vi "Split Bank DIO.vi"(0 "IN 19:0":fxp<+,20,20> format="%.0b") -> (2 "OUT 1:0":fxp<+,2,2>, 3 "OUT 3:2":fxp<+,2,2>, 4 "OUT 7:4":fxp<+,4,4>, 6 "OUT 9:8":fxp<+,2,2>, 8 "OUT 11:10":fxp<+,2,2>, 10 "OUT 13:12":fxp<+,2,2>, 13 "OUT 19:18":fxp<+,2,2>, 14 "OUT 17:16":fxp<+,2,2>, 15 "OUT 15:14":fxp<+,2,2>)   [LabVIEW 2021]
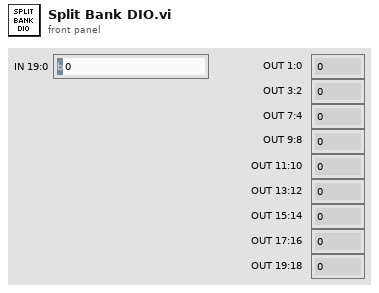
[diagram p1: front panel]
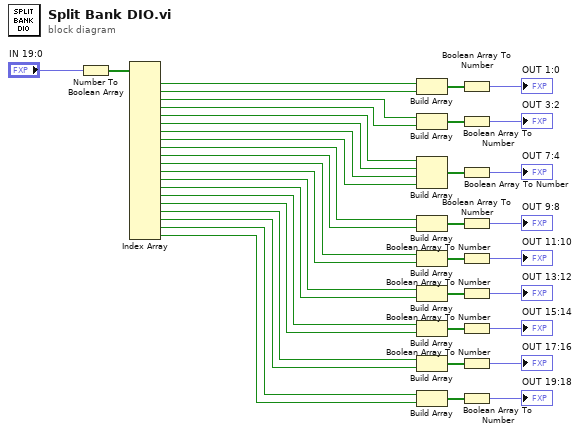
[diagram p0: block diagram]
diagram:
  n1 = Number To Boolean Array(number="IN 19:0") -> (Boolean array=w39:bool[])
  n2 = Index Array(array=w39) -> (element #1=w20:bool, element #2=w19:bool, element #3=w18:bool, element #4=w17:bool, element #5=w16:bool, element #6=w15:bool, element #7=w14:bool, element #8=w13:bool, element #9=w12:bool, element #10=w11:bool, element #11=w10:bool, element #12=w9:bool, element #13=w8:bool, element #14=w7:bool, element #15=w6:bool, element #16=w5:bool, element #17=w4:bool, element #18=w3:bool, element #19=w2:bool, element #20=w1:bool)  [unwired: 20 in]
  n3 = Build Array(w20, w19) -> (w38:bool[])
  n4 = Build Array(w18, w17) -> (w36:bool[])
  n5 = Build Array(w16, w15, w14, w13) -> (w35:bool[])
  n6 = Build Array(w12, w11) -> (w34:bool[])
  n7 = Build Array(w10, w9) -> (w33:bool[])
  n8 = Build Array(w8, w7) -> (w32:bool[])
  n9 = Build Array(w6, w5) -> (w31:bool[])
  n10 = Build Array(w4, w3) -> (w30:bool[])
  n11 = Build Array(w2, w1) -> (w29:bool[])
  n12 = Boolean Array To Number(Boolean array=w38) -> (number=→"OUT 1:0":fxp<+,2,2>)
  n13 = Boolean Array To Number(Boolean array=w36) -> (number=→"OUT 3:2":fxp<+,2,2>)
  n14 = Boolean Array To Number(Boolean array=w35) -> (number=→"OUT 7:4":fxp<+,4,4>)
  n15 = Boolean Array To Number(Boolean array=w34) -> (number=→"OUT 9:8":fxp<+,2,2>)
  n16 = Boolean Array To Number(Boolean array=w33) -> (number=→"OUT 11:10":fxp<+,2,2>)
  n17 = Boolean Array To Number(Boolean array=w32) -> (number=→"OUT 13:12":fxp<+,2,2>)
  n18 = Boolean Array To Number(Boolean array=w31) -> (number=→"OUT 15:14":fxp<+,2,2>)
  n19 = Boolean Array To Number(Boolean array=w30) -> (number=→"OUT 17:16":fxp<+,2,2>)
  n20 = Boolean Array To Number(Boolean array=w29) -> (number=→"OUT 19:18":fxp<+,2,2>)
